vi "Close Std In.vi"(8 "error in":errorcluster, 11 "ASE Handle":refnum<class "ase.lvclass">) -> (0 "error out":errorcluster, 1 "State":T1, 3 "ASE Handle Duplicate":refnum<class "ase.lvclass">)   [LabVIEW 2020, in "ase.lvlib" / "ase.lvclass"]
doc: "<B>Close the Standard Input.</B>\n\nThis will prevent any further writing to the standard input.\n\n<B>This VI will still operate when there is an error at the error-in terminal.</B>\n\nThis VI generates the following errors:\n-5691000: Internal Library Error. Check Error Message for more details.\n1556: Invalid Handle Supplied"
uses:
  ase.lvclass
  ase.lvclass/ase.ctl
  Standard Input State.ctl
  bin/ase_32-3.dll
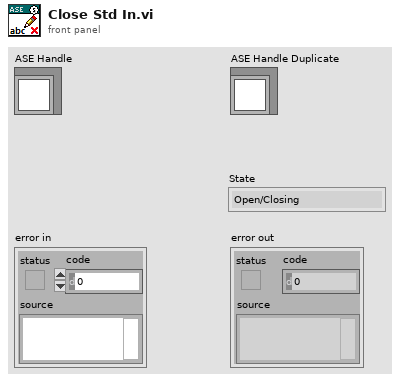
[diagram p1: front panel]
types:
  T1 = typedef "ase.lvlib/ase.lvclass/Standard Input State.ctl" = enum16{"Open/Closing", "Closed"}
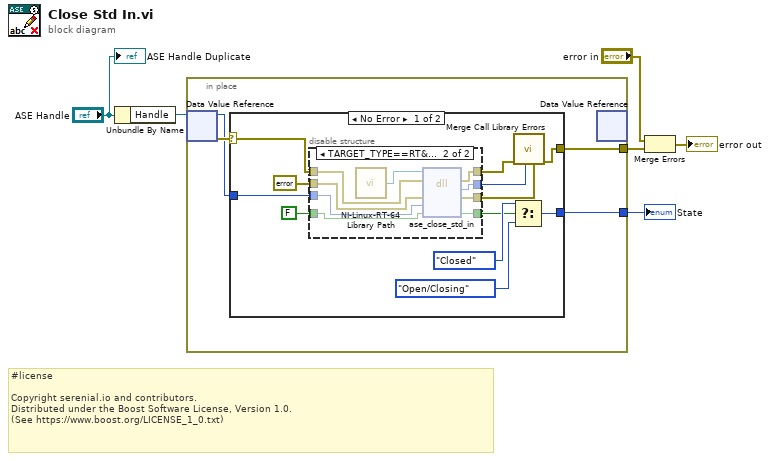
[diagram p0: block diagram]
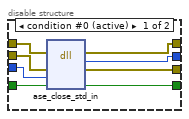
[diagram p2: hidden frame]
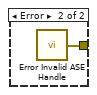
[diagram p3: hidden frame]
diagram:
  # "#license\n\nCopyright serenial.io and contributors.\nDistributed under the Boost Software License, Version 1.0.\n(See https://www.boost.org/LICENSE_1_0.txt)"
  n1 = Unbundle By Name("ASE Handle") -> ("Handle"=w3:refnum<data-value>)
  n2 = in-place "In Place Element Structure" {
    in-place-border: [w9] -> w6
    in-place-border: [w8] -> w4
    n3 = in-place-dvr #1(w3) -> (w7:u64, w10:errorcluster)
    n4 = case shown="No Error" w10 {
      selector: w10 -> [w11 _]
      tunnel: w7 -> [w17 _]
      tunnel: [w22 w40] -> w9
      tunnel: [w19 _] -> w8
      frame No Error {
        n5 = disable-structure shown="TARGET_TYPE==RT&&OS==Linux" {
          disable-tunnel: errorcluster {"status"=FALSE, "code"=0, "source"=""} ("error") -> [w29 w38]
          disable-tunnel: w17 -> [w28 w36]
          disable-tunnel: FALSE -> [w27 w35]
          disable-tunnel: [w23 w32] -> w15
          disable-tunnel: [w24 w33] -> w14
          disable-tunnel: [w25 w31] -> w13
          disable-tunnel: [w26 w34] -> w12
          disable-tunnel: w11 -> [w30 w37]
          frame condition #0 (active) {
            n6 = dll-call lib="C:/serenial/lib/asynchronous-system-exec/LabVIEW/ase/ase/bin/ase_*-3.*" fn="ase_close_std_in" ("AsyncSystemExec*.*:wrapperVersion")(error in=w30, "Error Out"=w29, "process"=w28, "already_closed"=w27) -> (error out=w23:errorcluster, "Error Code"=w24:i32, "Error Out"=w25:errorcluster, "already_closed"=w26:bool)  [unwired: 3 in, 1 out]
          }
          frame condition #1 {
            n7 = call "NI-Linux-RT-64 Library Path.vi"() -> ("Path"=w39:path)
            n8 = dll-call lib="?" fn="ase_close_std_in" ("AsyncSystemExec*.*:wrapperVersion")(path in=w39, error in=w37, "Error Out"=w38, "process"=w36, "already_closed"=w35) -> (error out=w32:errorcluster, "Error Code"=w33:i32, "Error Out"=w31:errorcluster, "already_closed"=w34:bool)  [unwired: 2 in, 1 out]
          }
        }
        n9 = Select(t=Standard_Input_State."Closed", s=w12, f=Standard_Input_State."Open/Closing" ("State")) -> (s? t:f=w19:T1)
        n10 = call "Merge Call Library Errors.vi"("Library Call Returned Error"=w13, "Error Code"=w14, "error in"=w15) -> ("error IO"=w22:errorcluster)  [unwired: 8 in]
      }
      frame Error {
        n11 = call "Error Invalid ASE Handle.vi"() -> ("Invalid ASE Handle"=w40:errorcluster)
      }
    }
    n12 = in-place-dvr #1() -> ()  [unwired: 1 in, 2 out]
  }
  "State" <- w4
  n13 = Merge Errors("error in", w6) -> (→"error out":errorcluster)
  "ASE Handle Duplicate" <- "ASE Handle"
